vi "Get Mandatory Objects.vi"(11 "EDS in":refnum<class "EDS.lvclass">) -> (2 "Mandatory Objects":refnum<class "Mandatory Objects.lvclass">, 3 "EDS out":refnum<class "EDS.lvclass">)   [LabVIEW 2024, in "EDS.lvlib" / "EDS.lvclass"]
uses:
  EDS.lvclass
  EDS.lvclass/EDS.ctl
  Mandatory Objects/Mandatory Objects.lvclass
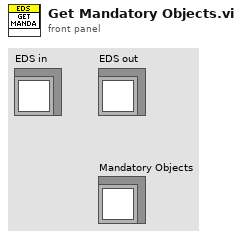
[diagram p1: front panel]
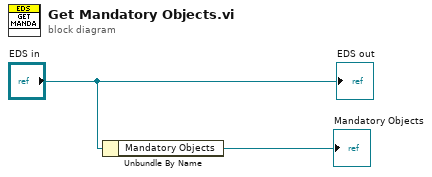
[diagram p0: block diagram]
diagram:
  n1 = Unbundle By Name("EDS in") -> ("Mandatory Objects"=→"Mandatory Objects":refnum<class "Mandatory Objects.lvclass">)
  "EDS out" <- "EDS in"
